vi "Distance Logger.vi"() -> ()   [LabVIEW 2011]
uses:
  Robot Global Data.vi
panel:
  out "Distance to Target":dbl[](graph)
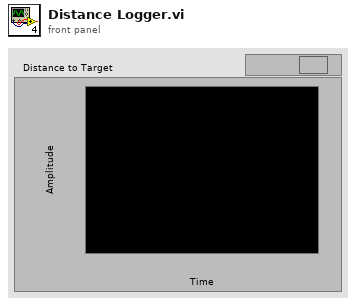
[diagram p1: front panel]
types:
  T1 = enum16{"open", "replace", "create", "open or create", "replace or create", "replace or create with confirmation"}
  T2 = cluster{"Position":cluster{"X":dbl, "Y":dbl}, "Distance (ft)":dbl}[]
  T3 = cluster{"Position":cluster{"X":dbl, "Y":dbl}, "Distance (ft)":dbl}
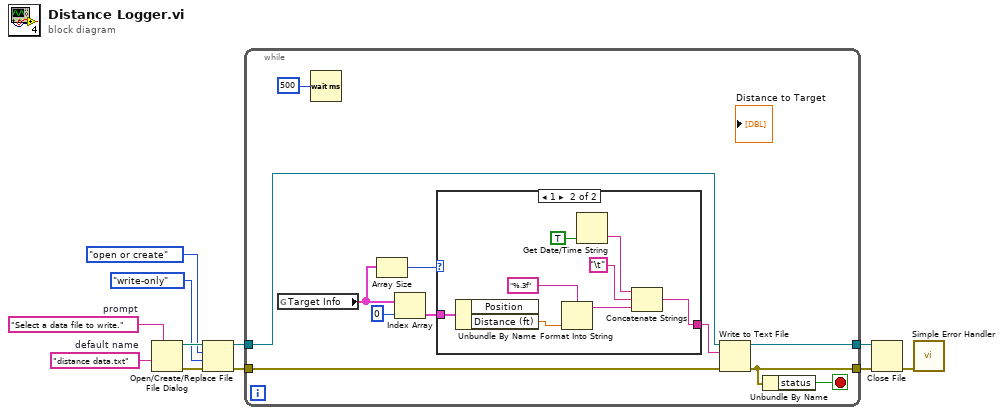
[diagram p0: block diagram]
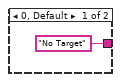
[diagram p2: hidden frame]
diagram:
  w10 = "distance data.txt"  # default name
  w9 = "Select a data file to write."  # prompt
  n1 = File Dialog(7:w9, 9:w10) -> (0:w8:errorcluster, 3:w11:path)  [unwired: 1 in, 6 out]
  n2 = Open/Create/Replace File(file path (use dialog)=w11, error in=w8, operation (0:open)=T1."open or create", access (0:read/write)=enum16{"read/write", "read-only", "write-only"}."write-only") -> (refnum out=w5:refnum<file>, error out=w4:errorcluster)  [unwired: 3 out]
  n3 = while {
    tunnel: w5 -> [w22]
    tunnel: w4 -> [w21]
    tunnel: [w20] -> w2
    tunnel: [w16] -> w1
    stop <- w15 stop-if-true
    n4 = global read "Robot Global Data.vi" "Target Info"() -> (w14:T2)
    n5 = Wait (ms)(milliseconds to wait=u32 500 ("millisecond multiple")) -> ()  [unwired: 1 out]
    n6 = Array Size(array=w14) -> (size(s)=w18:i32)
    n7 = Index Array(array=w14, index=0) -> (element=w12:T3)
    n8 = case shown="1" w18 {
      tunnel: ["No Target" w24] -> w17
      tunnel: w12 -> [_ w31]
      frame 0, Default {
      }
      frame 1 {
        n9 = Unbundle By Name(w31) -> ("Distance (ft)"=w30:dbl)  [unwired: 1 out]
        n10 = Format Into String(format string="%.3f", w30) -> (resulting string=w25:string)  [unwired: 2 in, 1 out]
        n11 = Get Date/Time String(want seconds? (F)=TRUE) -> (time string=w27:string)  [unwired: 2 in, 1 out]
        n12 = Concatenate Strings(w27, "\t", w25) -> (w24:string)
      }
    }
    n13 = Write to Text File(file (use dialog)=w22, text=w17, error in=w21) -> (refnum out=w20:refnum<file>, error out=w16:errorcluster)  [unwired: 1 in, 1 out]
    n14 = Unbundle By Name(w16) -> ("status"=w15:bool)
  }
  n15 = Close File(refnum=w2, error in=w1) -> (error out=w3:errorcluster)  [unwired: 1 out]
  n16 = call <vilib>:"Simple Error Handler.vi"("error in (no error)"=w3) -> ()  [unwired: 1 in, 8 out]
